vi "Resize Backlog.vi"(10 "Backlog Size":i32, 11 "ConsoleView Sink in":refnum<class "ConsoleView.lvclass">) -> (0 "error out":errorcluster, 3 "ConsoleView Sink out":refnum<class "ConsoleView.lvclass">)   [LabVIEW 2017, in "ConsoleView.lvlib" / "ConsoleView.lvclass"]
uses:
  ConsoleView.lvclass
  ConsoleView.lvclass/ConsoleView.ctl
  Composed Log/Types/Log Packet.ctl
  Composed Log/Types/Log Level.ctl
  Composed Log/Composed Log.lvlib
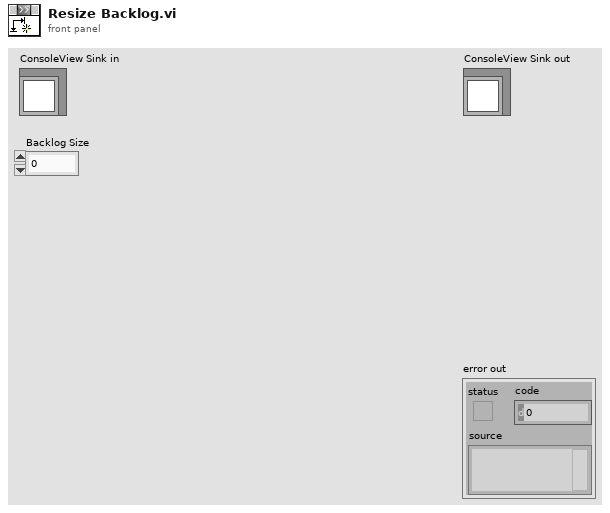
[diagram p1: front panel]
types:
  T1 = typedef "Composed Log.lvlib/Log Packet.ctl" = cluster{"Data To Log":string, "Source":string, "Event Level":T2, "Event Time":timestamp}
  T2 = typedef "Composed Log.lvlib/Log Level.ctl" = enum16{"Debug", "Info", "Warning", "Error", "Critical"}
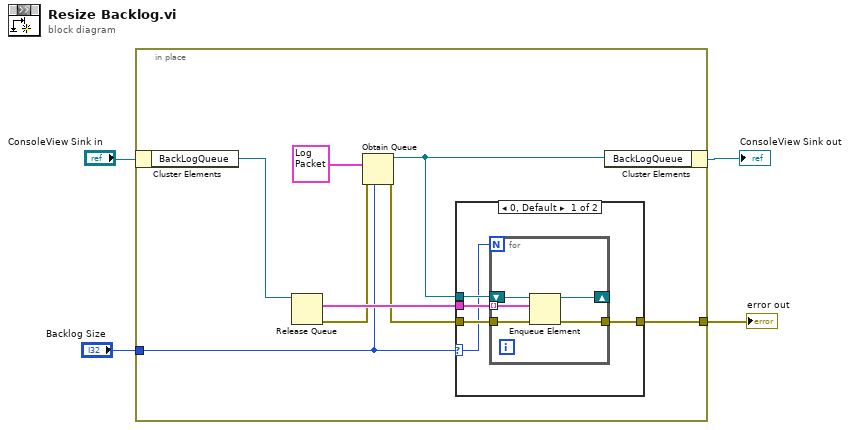
[diagram p0: block diagram]
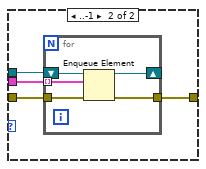
[diagram p2: hidden frame]
diagram:
  n1 = in-place {
    in-place-border: "Backlog Size" -> [w10]
    in-place-border: [w8] -> w3
    n2 = in-place-cluster #1("ConsoleView Sink in") -> ("BackLogQueue"=w6:refnum<queue>)
    n3 = Release Queue(queue=w6) -> (remaining elements=w12:T1[], error out=w7:errorcluster)  [unwired: 2 in, 1 out]
    n4 = Obtain Queue(max queue size (-1, unlimited)=w10, element data type=T1 {"Data To Log"="", "Source"="", "Event Level"=enum."Debug", "Event Time"=timestamp(0 s since 1904-01-01)} ("Log Packet"), error in (no error)=w7) -> (queue out=w5:refnum<queue>, error out=w11:errorcluster)  [unwired: 2 in, 1 out]
    n5 = case shown="0, Default" w10 {
      selector: w10 -> [w13 _]
      tunnel: w5 -> [w17 w26]
      tunnel: w12 -> [w16 w25]
      tunnel: [w14 w24] -> w8
      tunnel: w11 -> [w15 w23]
      frame 0, Default {
        n6 = for {
          N: w13 -> [_]
          tunnel: w16 -> [w18] mode=indexing
          shift-right: [w21] -> _
          shift-left: w17 -> [w22]
          tunnel: [w20] -> w14
          tunnel: w15 -> [w19]
          n7 = Enqueue Element(queue=w22, element=w18, error in (no error)=w19) -> (queue out=w21:refnum<queue>, error out=w20:errorcluster)  [unwired: 1 in, 1 out]
        }
      }
      frame ..-1 {
        n8 = for {
          tunnel: w25 -> [w27] mode=indexing
          shift-right: [w30] -> _
          shift-left: w26 -> [w31]
          tunnel: [w29] -> w24
          tunnel: w23 -> [w28]
          n9 = Enqueue Element(queue=w31, element=w27, error in (no error)=w28) -> (queue out=w30:refnum<queue>, error out=w29:errorcluster)  [unwired: 1 in, 1 out]
        }
      }
    }
    n10 = in-place-cluster #1("BackLogQueue"=w5) -> (→"ConsoleView Sink out":refnum<class "ConsoleView.lvclass">)
  }
  "error out" <- w3
